vi "Scale GUI.vi"(0 "Clust Refnum":refnum<vi>) -> ()   [LabVIEW 2012]
uses:
  DAQ configuration/scale type.ctl
  correspondence table.ctl
  pH/pH scale.ctl
  Dissolved Oxygen/DO scale.ctl
panel:
  out "size(s)":i32
  # "C"
  # "kPa"
  # "C"
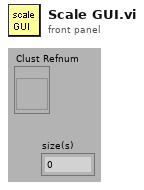
[diagram p1: front panel]
types:
  T1 = typedef "scale type.ctl" = enum16{"Volts", "Polynomial", "Correspondence Table", "pH", "Dissolved Oxygen", "Quadratic"}
  T2 = typedef "correspondence table.ctl" = cluster{"physical units":dbl, "volts":dbl}[]
  T3 = typedef "pH scale.ctl" = cluster{"Buffers":cluster{"Buffer":dbl, "Calibrated":bool, "V/T":dbl}[], "Temperature":dbl}
  T4 = typedef "DO scale.ctl" = cluster{"Temperature":dbl, "K":dbl, "barometric pressure":dbl}
  T5 = cluster{"conversion matrix":sgl[][], "units":string, "name":string, "scale type":T1, "offset (volts)":dbl, "second channel":i8, "correspondence table":T2, "offset (physical units)":dbl, "pH scale":T3, "D.O.":T4}
  T6 = cluster{"Controls[][0]":refnum<vi>, "Controls[][1]":refnum<vi>, "Controls[][2]":refnum<vi>, "Controls[][3]":refnum<vi>, "Controls[][4]":refnum<vi>, "Controls[][5]":refnum<vi>, "Controls[][6]":refnum<vi>, "Controls[][7]":refnum<vi>, "Controls[][8]":refnum<vi>, "Controls[][9]":refnum<vi>}
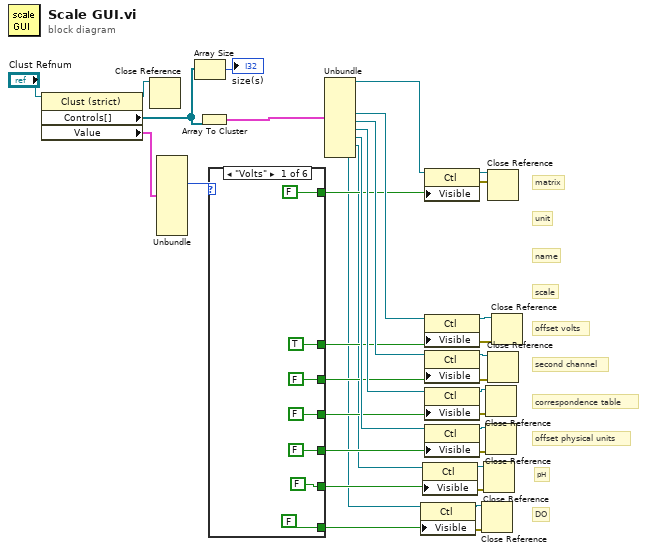
[diagram p0: block diagram]
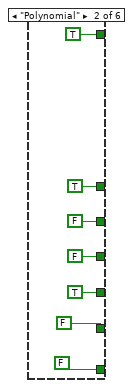
[diagram p2: hidden frame]
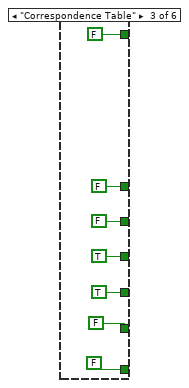
[diagram p3: hidden frame]
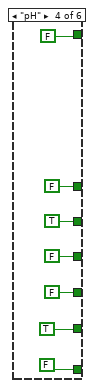
[diagram p4: hidden frame]
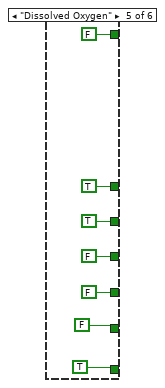
[diagram p5: hidden frame]
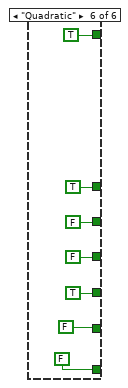
[diagram p6: hidden frame]
diagram:
  # "DO"
  # "pH"
  # "offset physical units"
  # "correspondence table"
  # "second channel"
  # "offset volts"
  # "scale"
  # "name"
  # "unit"
  # "matrix"
  n1 = property class="Clust (strict)"(reference="Clust Refnum") -> (reference out=w20:refnum<vi>, "Controls[]"=w33:refnum<vi>[], "Value"=w35:T5)  [unwired: 1 in, 1 out]
  n2 = Close Reference(reference=w20) -> ()  [unwired: 1 in, 1 out]
  n3 = Unbundle(w35) -> ("scale type"=w34:T1)  [unwired: 9 out]
  n4 = Array Size(array=w33) -> (size(s)=→"size(s)":i32)
  n5 = Array To Cluster(array=w33) -> (cluster=w31:T6)
  n6 = case shown="\"Volts\"" w34 {
    tunnel: [TRUE TRUE FALSE FALSE TRUE TRUE] -> w25
    tunnel: [FALSE FALSE FALSE TRUE TRUE FALSE] -> w24
    tunnel: [FALSE FALSE TRUE FALSE FALSE FALSE] -> w23
    tunnel: [FALSE TRUE TRUE FALSE FALSE TRUE] -> w22
    tunnel: [FALSE TRUE FALSE FALSE FALSE TRUE] -> w21
    tunnel: [FALSE FALSE FALSE TRUE FALSE FALSE] -> w7
    tunnel: [FALSE FALSE FALSE FALSE TRUE FALSE] -> w3
    frame "Volts" {
    }
    frame "Polynomial" {
    }
    frame "Correspondence Table" {
    }
    frame "pH" {
    }
    frame "Dissolved Oxygen" {
    }
    frame "Quadratic" {
    }
  }
  n7 = Unbundle(w31) -> ("Controls[][0]"=w30:refnum<vi>, "Controls[][4]"=w29:refnum<vi>, "Controls[][5]"=w28:refnum<vi>, "Controls[][6]"=w27:refnum<vi>, "Controls[][7]"=w26:refnum<vi>, "Controls[][8]"=w8:refnum<vi>, "Controls[][9]"=w4:refnum<vi>)  [unwired: 3 out]
  n8 = property class="Ctl"(reference=w4, "Visible"=w3) -> (reference out=w2:refnum<vi>, error out=w5:errorcluster)  [unwired: 1 in]
  n9 = property class="Ctl"(reference=w8, "Visible"=w7) -> (reference out=w6:refnum<vi>, error out=w9:errorcluster)  [unwired: 1 in]
  n10 = property class="Ctl"(reference=w30, "Visible"=w21) -> (reference out=w11:refnum<vi>, error out=w10:errorcluster)  [unwired: 1 in]
  n11 = property class="Ctl"(reference=w29, "Visible"=w25) -> (reference out=w18:refnum<vi>, error out=w19:errorcluster)  [unwired: 1 in]
  n12 = property class="Ctl"(reference=w28, "Visible"=w24) -> (reference out=w16:refnum<vi>, error out=w17:errorcluster)  [unwired: 1 in]
  n13 = property class="Ctl"(reference=w27, "Visible"=w23) -> (reference out=w14:refnum<vi>, error out=w15:errorcluster)  [unwired: 1 in]
  n14 = property class="Ctl"(reference=w26, "Visible"=w22) -> (reference out=w12:refnum<vi>, error out=w13:errorcluster)  [unwired: 1 in]
  n15 = Close Reference(reference=w2, error in (no error)=w5) -> ()  [unwired: 1 out]
  n16 = Close Reference(reference=w6, error in (no error)=w9) -> ()  [unwired: 1 out]
  n17 = Close Reference(reference=w14, error in (no error)=w15) -> ()  [unwired: 1 out]
  n18 = Close Reference(reference=w12, error in (no error)=w13) -> ()  [unwired: 1 out]
  n19 = Close Reference(reference=w11, error in (no error)=w10) -> ()  [unwired: 1 out]
  n20 = Close Reference(reference=w16, error in (no error)=w17) -> ()  [unwired: 1 out]
  n21 = Close Reference(reference=w18, error in (no error)=w19) -> ()  [unwired: 1 out]
